vi "MeasureDC.vi"() -> ()   [LabVIEW 2011]
panel:
  out "return":i32
  in  "stop":bool
  out "Displayed Hologram":u8[][](graph)
  in  "N_iterations":i32=10
  in  "e_desired":sgl=1.0
  in  "TrueFrame":i32=3
  in  "deviceId":i32
  in  "Path to LUT file":path
  in  "SLM enabled":bool
  in  "Grid spacing":i32=8
  in  "Spots y":i32=3
  in  "Spots x":i32=3
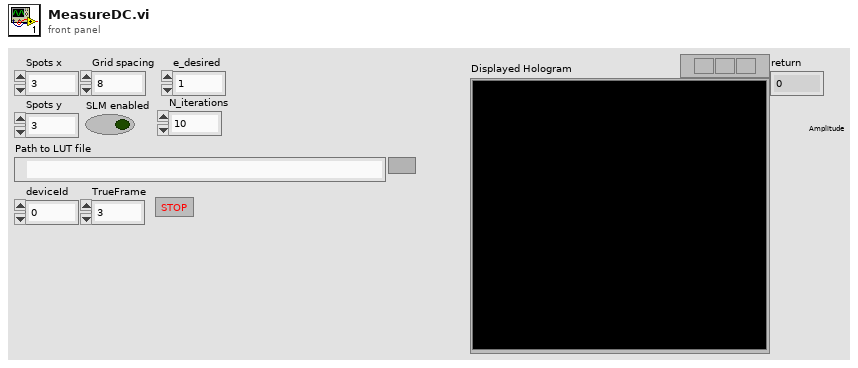
[diagram p1: front panel]
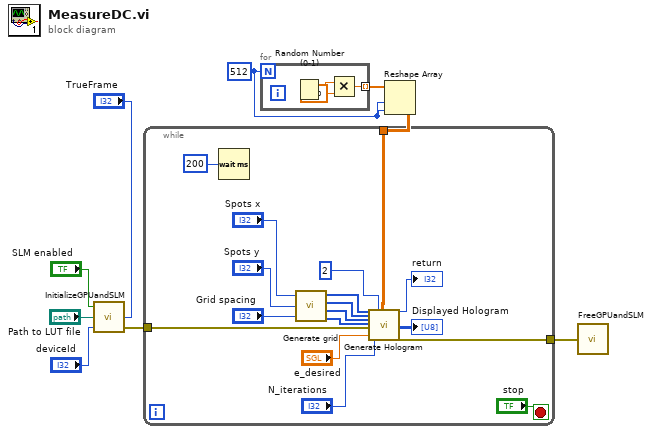
[diagram p0: block diagram]
diagram:
  w1 = 512
  n1 = call "InitializeGPUandSLM.vi"("TrueFrame"="TrueFrame", "deviceId"="deviceId", "Path to LUT file"="Path to LUT file", "SLM enabled"="SLM enabled") -> ("CUDA/SLM error"=w5:errorcluster)  [unwired: 1 out]
  n2 = for {
    N: w1 -> [_]
    tunnel: [w10] -> w3 mode=indexing
    n3 = Random Number (0-1)() -> (number: 0 to 1=w12:dbl)
    n4 = Multiply(x=w12, y=255.0) -> (x*y=w10:dbl)
  }
  n5 = Reshape Array(w3, w1, w1) -> (w2:dbl[][])
  n6 = while {
    tunnel: w5 -> [w19]
    tunnel: [w16] -> w4
    tunnel: w2 -> [w13]
    stop <- "stop" stop-if-true
    n7 = Wait (ms)(milliseconds to wait=u32 200) -> ()  [unwired: 1 out]
    n8 = call "Generate grid.vi"("Spots x"="Spots x", "Spots y"="Spots y", "Grid spacing"="Grid spacing") -> ("X"=w26:i32[], "Y"=w25:i32[], "Z"=w24:i32[], "A"=w23:i32[])
    n9 = call "Generate Hologram.vi"("x"=w26, "y"=w25, "z"=w24, "spot_intensities"=w23, "CUDA/SLM error in"=w19, "e_desired"="e_desired", "N_iterations"="N_iterations", "method"=2, "CGH in"=w13) -> ("return"=→"return":i32, "CGH out"=→"Displayed Hologram":u8[][], "CUDA/SLM error out"=w16:errorcluster)  [unwired: 15 in, 1 out]
  }
  n10 = call "FreeGPUandSLM.vi"("error in"=w4) -> ()  [unwired: 2 out]
